vi "Template Files List.vi"() -> (2 "template files":string[](array[string])=["Measurement Configuration.ctl", "Measurement Results.ctl", "Create Measurement.vi", "Start Measurement.vi", "Read Measurement.vi", "Run Client.vi"])   [LabVIEW 2021, in "NI Measurement V2 Client Generator Runtime.lvlib"]
uses:
  NI Measurement V2 Client Generator Runtime.lvlib
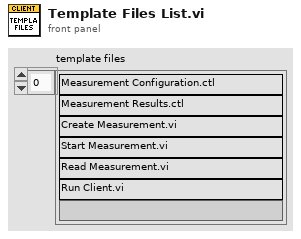
[diagram p1: front panel]
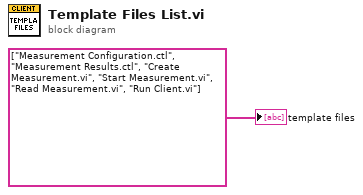
[diagram p0: block diagram]
diagram:
  "template files" <- string[] ["Measurement Configuration.ctl", "Measurement Results.ctl", "Create Measurement.vi", "Start Measurement.vi", "Read Measurement.vi", "Run Client.vi"]
